vi "MB_C843.21_init_mod.vi"(6 "Limit switch selection":u16(ring) items=["Positive (FPL)", "Negative (FNL)"], 8 "error in":errorcluster, 9 "USB settings":cluster{"S/N":string, "USB Search?":bool}={"S/N"="", "USB Search?"=TRUE}, 10 "RON settings":T1={"RON Affected axes"=[], "Reference mode"=[], "Check FRF?"=TRUE}, 11 "System no.":i32=1) -> (0 "error out":errorcluster, 1 "SN out":string, 2 "C863\nConn. \nAxis":string[](array[string]), 4 "Identification":string, 5 "+/- movement\nrange":dbl[](array[numeric]) format="%.6f")   [LabVIEW 2011]
panel:
  in  "All axes?":bool
  in  "Switch servo on?":bool=TRUE
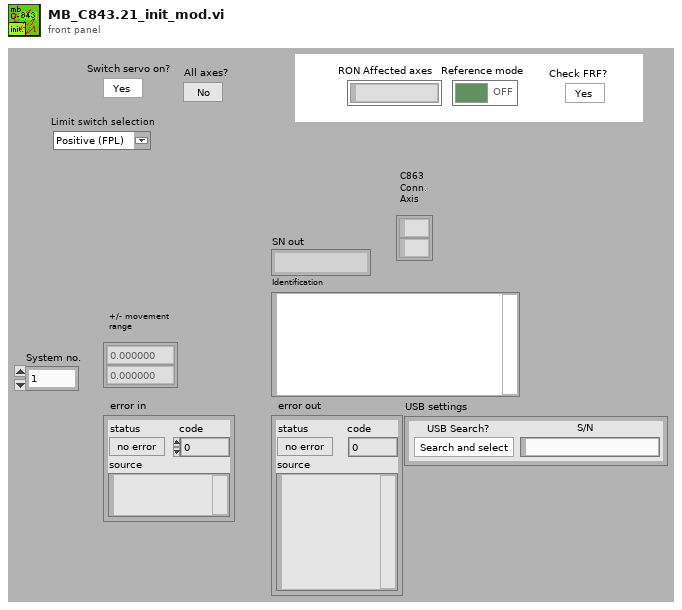
[diagram p1: front panel]
types:
  T1 = cluster{"RON Affected axes":string[], "Reference mode":bool[], "Check FRF?":bool}
  T2 = cluster{"Register DC":bool, "DaisyChain Search?":bool, "Device ID":i32}
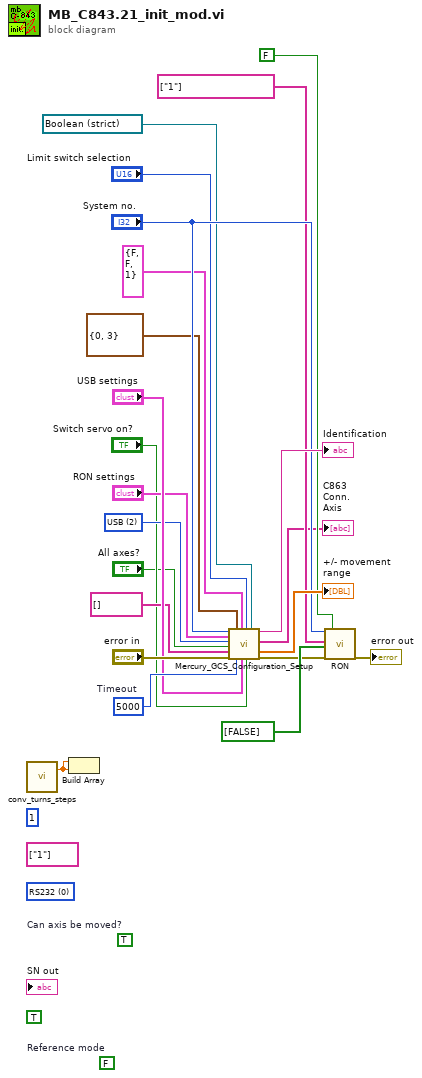
[diagram p0: block diagram]
diagram:
  (unwired) 1 ("Device ID out")
  w16 = u16 2 items=["RS232", "RS232 DaisyChain", "USB", "USB_DaisyChain"] ("Interface")
  (unwired) string[] ["1"] ("RON Affected axes")
  (unwired) TRUE
  (unwired) FALSE  # Reference mode
  (unwired) TRUE  # Can axis be moved?
  w22 = u32 5000  # Timeout
  (unwired) u16 0 items=["RS232", "USB"] ("Interface")
  n1 = call "conv_turns_steps.vi"() -> ("Steps(-)"=w13:dbl)  [unwired: 2 in, 1 out]
  n2 = Build Array(w13, w13) -> ()  [unwired: 1 out]
  n3 = call "Mercury_GCS_Configuration_Setup.vi"("System no."="System no.", "RON settings"="RON settings", "Interface"=w16, "All axes?"="All axes?", "Axes to move"=string[] [], "error in"="error in", "RS232 settings"=cluster{"Portnumber":i32, "Baudrate":u16} {"Portnumber"=0, "Baudrate"=3}, "Timeout"=w22, "DaisyChain settings"=T2 {"Register DC"=FALSE, "DaisyChain Search?"=FALSE, "Device ID"=1}, "USB settings"="USB settings", "Limit switch selection"="Limit switch selection", "Switch servo on?"="Switch servo on?", "Stop refnum"=refnum<vi> refnum) -> ("Identification"=→"Identification":string, "Conn. \nAxes"=→"C863\nConn. \nAxis":string[], "+/- movement\nrange"=→"+/- movement\nrange":dbl[], "error out"=w1:errorcluster)  [unwired: 3 out]
  n4 = call "RON.vi"("System no."="System no.", "Axes to command"=string[] ["1"] ("RON Affected axes"), "Reference mode"=bool[] [FALSE], "error in"=w1, "Without axis ID?"=FALSE) -> ("error out"=→"error out":errorcluster)  [unwired: 14 out]
